vi "Parse_GPGGA (SubVI).vi"(9 "Array":string[](array[string])) -> (0 "GPGGA?":bool, 2 "GPGGA array":string[](array[string]))   [LabVIEW 2017]
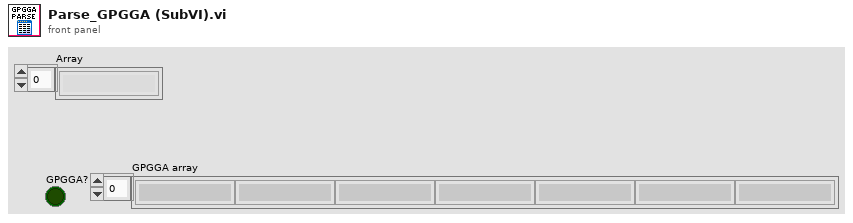
[diagram p1: front panel]
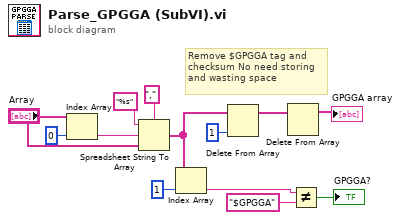
[diagram p0: block diagram]
diagram:
  # "Remove $GPGGA tag and \nchecksum No need storing and wasting space"
  n1 = Index Array(array="Array", index=0) -> (element=w10:string)
  n2 = Spreadsheet String To Array(delimiter (Tab)=",", format string="%s", spreadsheet string=w10, array type (2D Dbl)="Array") -> (array=w4:string[])
  n3 = Index Array(array=w4, index=1 ("disabled index (col)")) -> (element=w7:string)
  n4 = Delete From Array(array=w4, index=1) -> (array with subset deleted=w2:string[])  [unwired: 1 in, 1 out]
  n5 = Delete From Array(array=w2) -> (array with subset deleted=→"GPGGA array":string[])  [unwired: 2 in, 1 out]
  n6 = Not Equal?(x=w7, y="$GPGGA") -> (x != y?=→"GPGGA?":bool)
